vi "Ticks To Degrees.vi"(11 "Steer Angles (ticks)":T1) -> (3 "Steer Angles (degrees)":T1)   [LabVIEW 2020]
doc: "unit conversion: ticks --> degrees (cancoder units)"
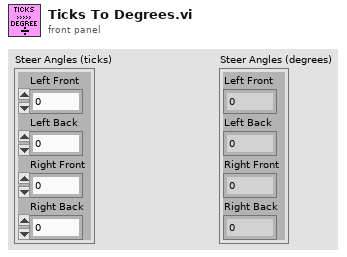
[diagram p1: front panel]
types:
  T1 = cluster{"Left Front":i32, "Left Back":i32, "Right Front":i32, "Right Back":i32}
  T2 = cluster{"Left Front":dbl, "Left Back":dbl, "Right Front":dbl, "Right Back":dbl}
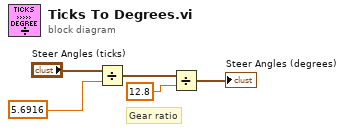
[diagram p0: block diagram]
diagram:
  # "Gear ratio"
  n1 = Divide(x="Steer Angles (ticks)", y=5.6916 ("Scale Factor")) -> (x/y=w5:T2)
  n2 = Divide(x=w5, y=12.8) -> (x/y=→"Steer Angles (degrees)":T2)
